vi "LDA_Align_PN_8 point.vi"(1 "Align Probe Using":enum16{"Green Beams", "Blue Beams"}(ring), 2 "Use Specification Beam Half-Angle":bool) -> (0 "Beam Data":T2={"Vg1 (Green 1 dir. vect.)"=[0.059117350659853476, -0.996541267827751, 0.05840068807144843], "Vg2  (Green 2 dir. vect.)"=[-0.05232536310393669, -0.9971561380468801, -0.054237373935992664], "Vb1 (Blue 1 dir. vect.)"=[-0.052923229613528855, -0.9969242065933935, 0.057803616456121795], "Vb2 (Blue 1 dir. vect.)"=[0.05971521716944564, -0.9967731992812374, -0.05364030232066602], "Porb (Orb XYZ posn. forced coplanar)"=[2201.0738225655555, -1199.3737231995547, 269.758310600838], "Porb (Orb XYZ posn. - allow skew)"=[2200.796256301178, -1199.3740953152687, 270.0329332816893], "Orb posn. uncertainty, +/- dx, dy, dz"=[0.13878313218879157, 0.00018605785703584843, 0.13731134042564008], "Vp (Actual Probe dir. vect)"=[0.003406702197773746, -0.9999920168246164, 0.0020882210543692924], "Yaw (deg)"=89.80480953887573, "Pitch (deg)"=0.11964634006213794, "In-Plane Roll (deg)"=45.305328966424156, "Beam Half Angle (deg)"=4.544091484248422, "B1 Close P11"=[0.0, 0.0, 0.0], "B1 Far P12"=[2158.01, -491.04, 229.28], "B2 Close P22"=[2158.01, -491.04, 229.28], "B2 Far P21"=[2158.01, -491.04, 229.28], "Projected Roll (deg)"=0.0, "Green Velocity Vector"=[0.0, 0.0, 0.0], "Blue Velocity Vector"=[0.0, 0.0, 0.0], "Probe is facing...."="-", "Calculation Method"=""} {"Vp (Actual Probe dir. vect)" format="%#_6f"; "Vg2  (Green 2 dir. vect.)" format="%#_6f"; "Vg1 (Green 1 dir. vect.)" format="%#_6f"})   [LabVIEW 2012]
uses:
  Controls/LDA_Beam_Cluster.ctl
  Gen Trav/Route mapping/Axis.ctl
  Controls/Tunnel_Coordinates.ctl
  Controls/Post_Process.ctl
  Controls/Setup.ctl
  Gen Trav/Trav_mode.ctl
  Controls/User_Specific_mode.ctl
  Globals/LDA_meas_global_1.vi
  Globals/Trav_pos_global.vi
panel:
  out "8 Peaked positions":dbl[][](array[numeric])
  out "Peakup up inputs":dbl[][](array[numeric])
  out "Fixed Axis":T1
  out "png folder":path
  out "Taught point names":string[](array[string])
  out "Taught Positions":dbl[][](array[numeric])
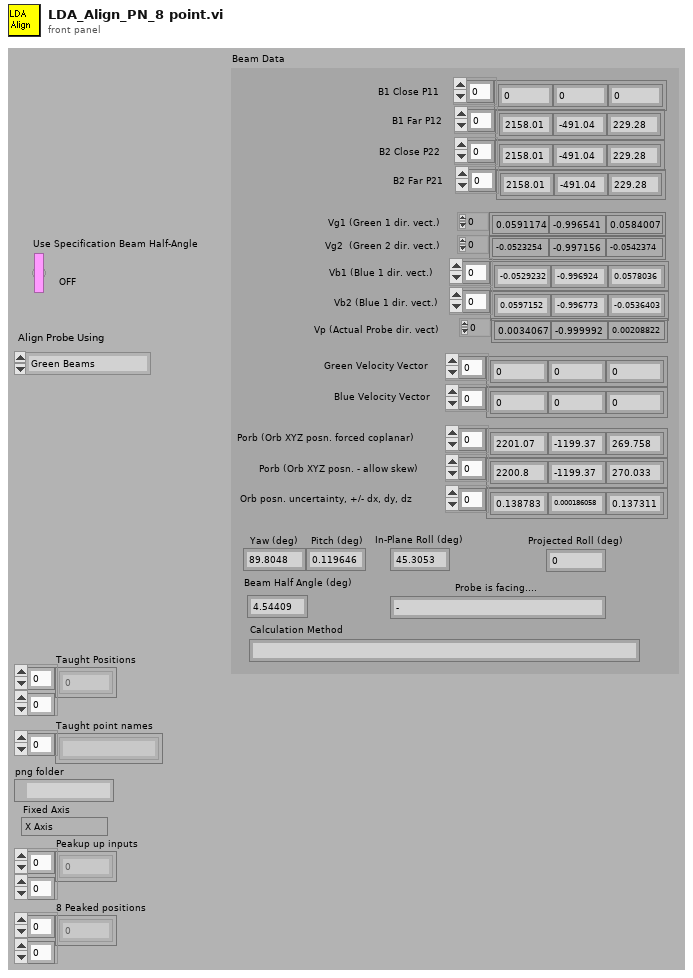
[diagram p1: front panel]
types:
  T1 = typedef "Axis.ctl" = enum16{"X Axis", "X Axis -ve", "Y Axis", "Y Axis -ve", "Z Axis", "Z Axis -ve"}
  T2 = typedef "LDA_Beam_Cluster.ctl" = cluster{"Vg1 (Green 1 dir. vect.)":dbl[], "Vg2  (Green 2 dir. vect.)":dbl[], "Vb1 (Blue 1 dir. vect.)":dbl[], "Vb2 (Blue 1 dir. vect.)":dbl[], "Porb (Orb XYZ posn. forced coplanar)":dbl[], "Porb (Orb XYZ posn. - allow skew)":dbl[], "Orb posn. uncertainty, +/- dx, dy, dz":dbl[], "Vp (Actual Probe dir. vect)":dbl[], "Yaw (deg)":dbl, "Pitch (deg)":dbl, "In-Plane Roll (deg)":dbl, "Beam Half Angle (deg)":dbl, "B1 Close P11":dbl[], "B1 Far P12":dbl[], "B2 Close P22":dbl[], "B2 Far P21":dbl[], "Projected Roll (deg)":dbl, "Green Velocity Vector":dbl[], "Blue Velocity Vector":dbl[], "Probe is facing....":string, "Calculation Method":string}
  T3 = typedef "Tunnel_Coordinates.ctl" = enum16{"Work in Tunnel Coordinates", "Work in Model Coordinates"}
  T4 = typedef "Setup.ctl" = enum16{"Run Program", "Show Setup", "Save Current Setup", "Setup Front Panel"}
  T5 = typedef "Post_Process.ctl" = enum16{"Take New Data", "Post Process Raw Data File"}
  T6 = typedef "User_Specific_mode.ctl" = enum16{"Check VI only", "Run VI"}
  T7 = typedef "Trav_mode.ctl" = enum16{"Move traverse", "Read traverse position", "Teach Position"}
  T8 = enum16{"Load setup from excel file", "Save setup to excel file"}
  T9 = cluster{"second":i32, "minute":i32, "hour":i32, "day of month":i32, "month":i32, "year":i32, "day of week":i32, "day of year":i32, "is DST":i32}
  T10 = typedef "Multi_Run_Status.ctl" = enum16{"Continue", "Jump to Next Point", "Jump to Next Row", "Jump To Fall Back", "Terminate Run"}
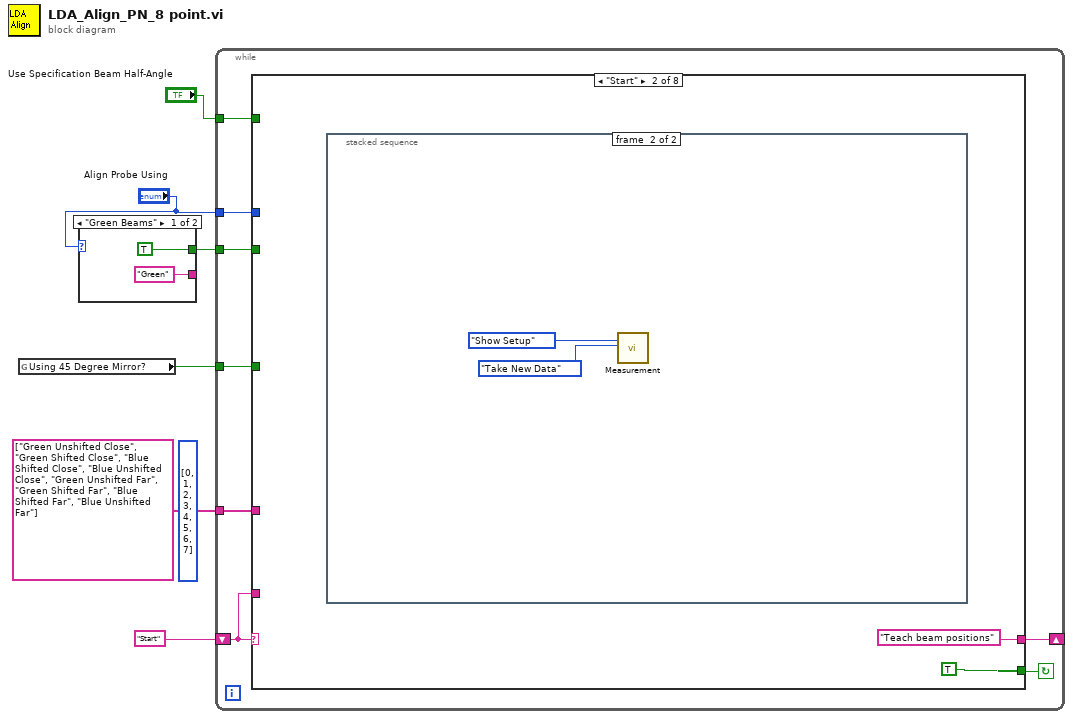
[diagram p0: block diagram]
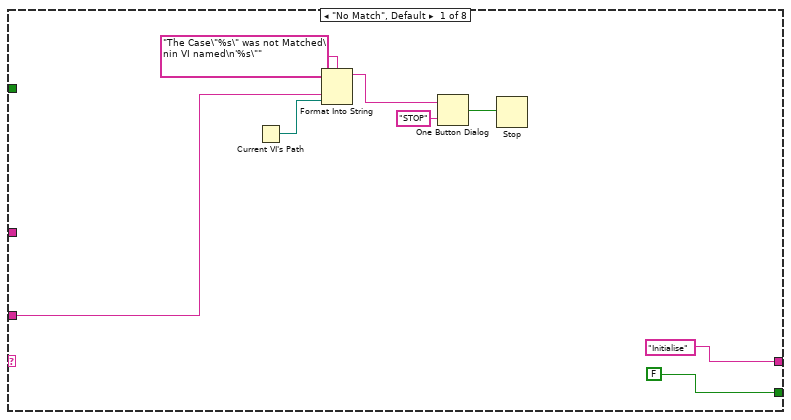
[diagram p2: hidden frame]
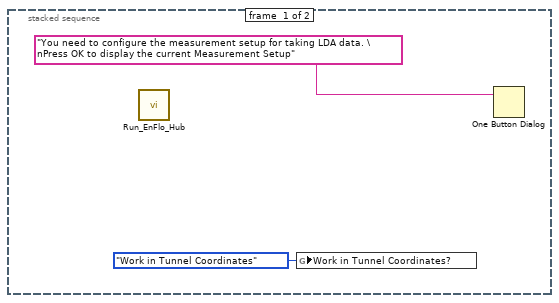
[diagram p3: hidden frame]
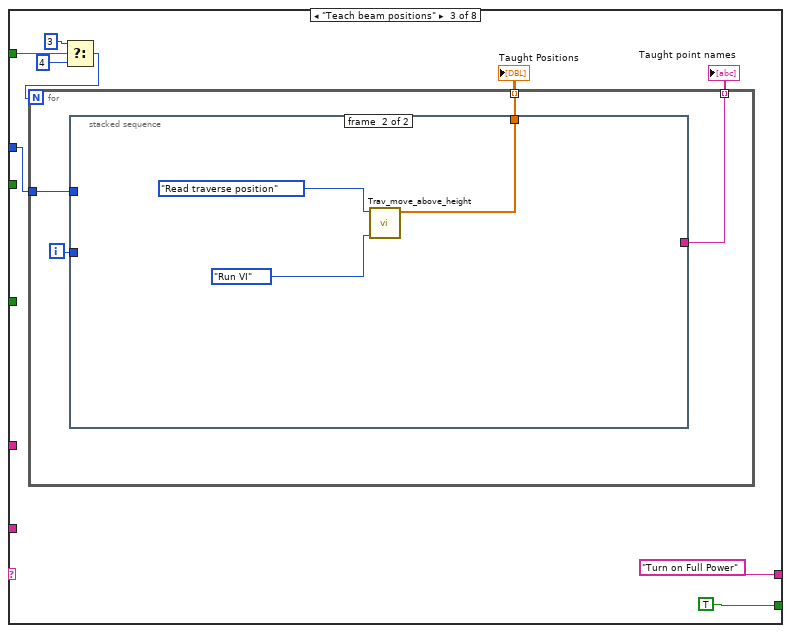
[diagram p4: hidden frame]
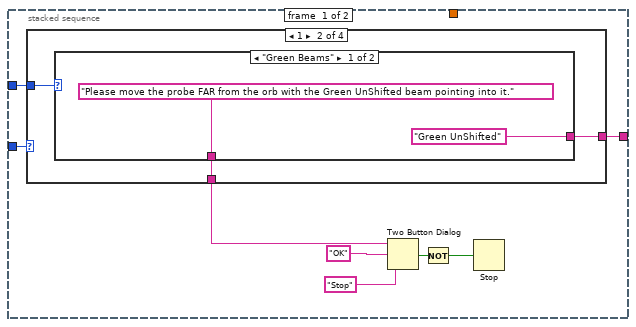
[diagram p5: hidden frame]
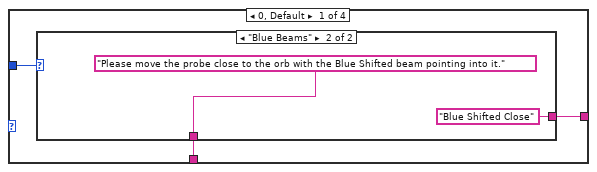
[diagram p6: hidden frame]
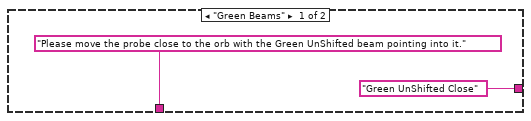
[diagram p7: hidden frame]
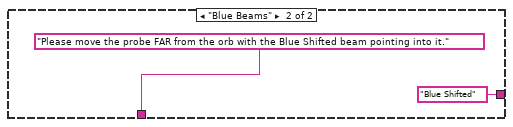
[diagram p8: hidden frame]
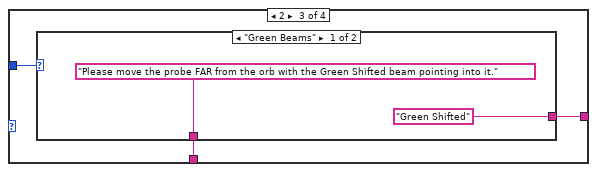
[diagram p9: hidden frame]
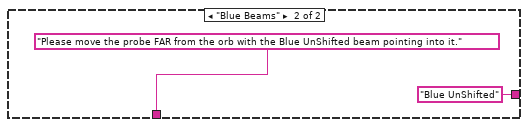
[diagram p10: hidden frame]
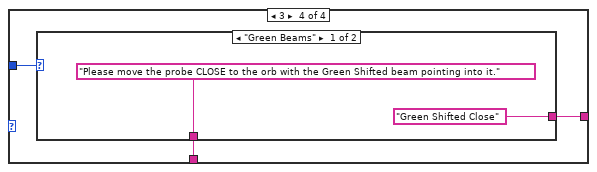
[diagram p11: hidden frame]
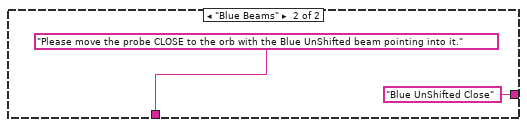
[diagram p12: hidden frame]
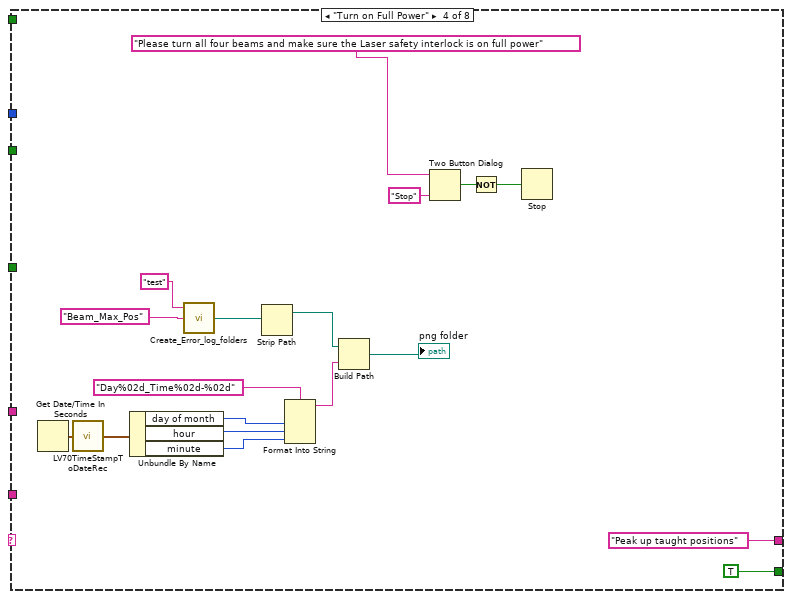
[diagram p13: hidden frame]
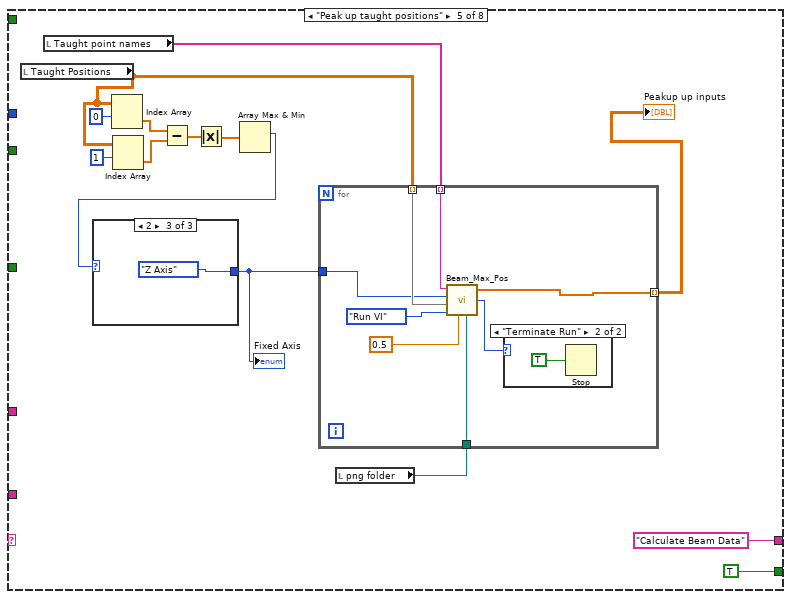
[diagram p14: hidden frame]
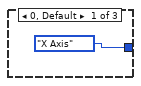
[diagram p15: hidden frame]
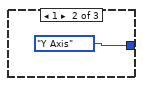
[diagram p16: hidden frame]
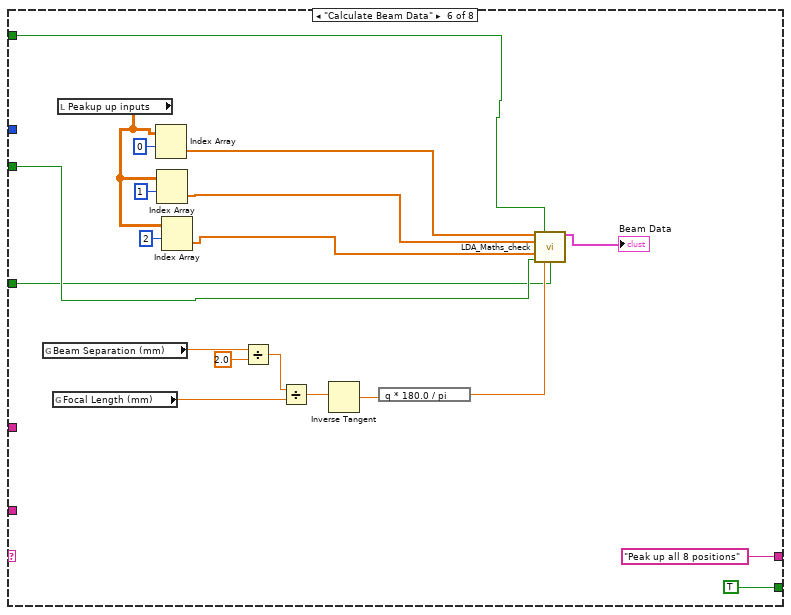
[diagram p18: hidden frame]
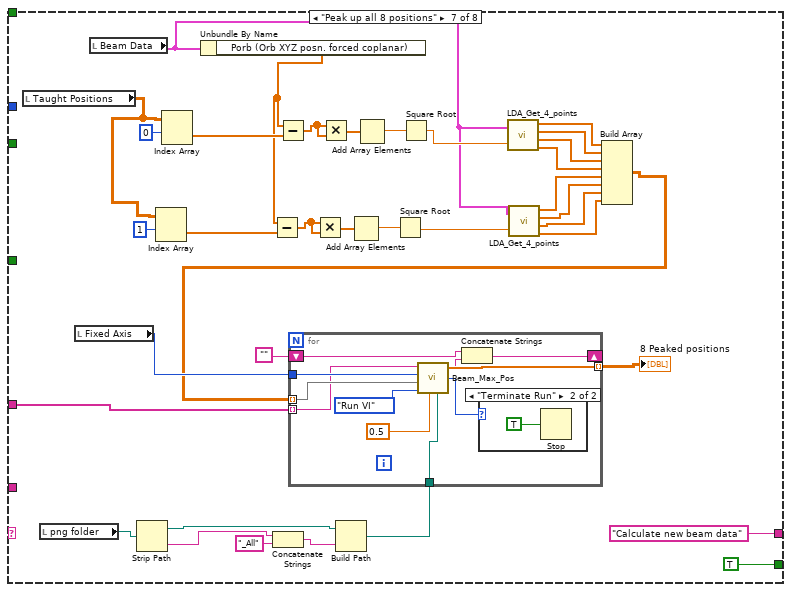
[diagram p19: hidden frame]
diagram:
  (unwired) i32[] [0, 1, 2, 3, 4, 5, 6, 7] ("appended array")
  n1 = global read "LDA_meas_global_1.vi" "Using 45 Degree Mirror?"() -> (w1:bool)
  n2 = case shown="\"Green Beams\"" "Align Probe Using" {
    tunnel: [TRUE FALSE] -> w3
    tunnel: ["Green" "Blue"] -> _
    frame "Green Beams" {
    }
    frame "Blue Beams" {
    }
  }
  n3 = while {
    shift-left: "Start" -> [w16]
    shift-right: [w17] -> _
    tunnel: "Align Probe Using" -> [w15]
    tunnel: "Use Specification Beam Half-Angle" -> [w14]
    tunnel: w3 -> [w13]
    tunnel: string[] ["Green Unshifted Close", "Green Shifted Close", "Blue Shifted Close", "Blue Unshifted Close", "Green Unshifted Far", "Green Shifted Far", "Blue Shifted Far", "Blue Unshifted Far"] ("appended array") -> [w12]
    tunnel: w1 -> [w11]
    stop <- w18 continue-if-true
    n4 = case shown="\"Start\"" w16 {
      tunnel: [FALSE TRUE TRUE TRUE TRUE TRUE TRUE FALSE] -> w18
      tunnel: ["Initialise" "Teach beam positions" "Turn on Full Power" "Peak up taught positions" "Calculate Beam Data" "Peak up all 8 positions" "Calculate new beam data" "Log Check Angles panel"] -> w17
      tunnel: w16 -> [w21 _ _ _ _ _ _ _]
      tunnel: w15 -> [_ _ w39 _ _ _ _ _]
      tunnel: w14 -> [_ _ w36 _ _ w146 _ _]
      tunnel: w13 -> [_ _ _ _ _ w145 _ _]
      tunnel: w12 -> [_ _ _ _ _ _ w151 _]
      tunnel: w11 -> [_ _ _ _ _ w129 _ w197]
      frame "No Match", Default {
        n5 = Current VI's Path() -> (path=w20:path)
        n6 = Format Into String(format string="The Case\"%s\" was not Matched\nin VI named\n'%s\"" ("Format String"), w21, w20) -> (resulting string=w24:string)  [unwired: 2 in, 1 out]
        n7 = One Button Dialog(message=w24, button name ("OK")="STOP") -> (true=w22:bool)
        n8 = Stop(stop? (T)=w22) -> ()
      }
      frame "Start" {
        n9 = stacked-sequence {
          frame #0 {
            n10 = call "Run_EnFlo_Hub.vi"() -> ()  [unwired: 8 out]
            n11 = global write "Trav_pos_global.vi" "Work in Tunnel Coordinates?"(Tunnel_Coordinates."Work in Tunnel Coordinates" ("Work in Tunnel Coordinates?")) -> ()
            n12 = One Button Dialog(message="You need to configure the measurement setup for taking LDA data. \nPress OK to display the current Measurement Setup") -> ()  [unwired: 1 in, 1 out]
          }
          frame #1 {
            n13 = call "Measurement.vi"("setup"=Setup."Show Setup", "Post Process"=Post_Process."Take New Data") -> ()  [unwired: 16 in, 2 out]
          }
        }
      }
      frame "Teach beam positions" {
        n14 = Select(t=3, s=w36, f=4) -> (s? t:f=w35:i32)
        n15 = for {
          N: w35 -> [_]
          tunnel: [w45] -> w34 mode=indexing
          tunnel: w39 -> [w44]
          tunnel: [w43] -> w33 mode=indexing
          i -> [w42]
          n16 = stacked-sequence {
            tunnel: [_ w82] -> w45
            tunnel: w44 -> [w52 _]
            tunnel: [w47 _] -> w43
            tunnel: w42 -> [w46 _]
            frame #0 {
              n17 = case shown="1" w46 {
                tunnel: [w56 w63 w70 w77] -> w53
                tunnel: w52 -> [w55 w62 w69 w76]
                tunnel: [w54 w61 w68 w75] -> w47
                frame 0, Default {
                  n18 = case shown="\"Blue Beams\"" w55 {
                    tunnel: ["Please move the probe close to the orb with the Green UnShifted beam pointing into it." ("message") "Please move the probe close to the orb with the Blue Shifted beam pointing into it." ("message")] -> w56
                    tunnel: ["Green UnShifted Close" "Blue Shifted Close"] -> w54
                    frame "Green Beams" {
                    }
                    frame "Blue Beams" {
                    }
                  }
                }
                frame 1 {
                  n19 = case shown="\"Green Beams\"" w62 {
                    tunnel: ["Please move the probe FAR from the orb with the Green UnShifted beam pointing into it." ("message") "Please move the probe FAR from the orb with the Blue Shifted beam pointing into it." ("message")] -> w63
                    tunnel: ["Green UnShifted" "Blue Shifted"] -> w61
                    frame "Green Beams" {
                    }
                    frame "Blue Beams" {
                    }
                  }
                }
                frame 2 {
                  n20 = case shown="\"Green Beams\"" w69 {
                    tunnel: ["Please move the probe FAR from the orb with the Green Shifted beam pointing into it." ("message") "Please move the probe FAR from the orb with the Blue UnShifted beam pointing into it." ("message")] -> w70
                    tunnel: ["Green Shifted" "Blue UnShifted"] -> w68
                    frame "Green Beams" {
                    }
                    frame "Blue Beams" {
                    }
                  }
                }
                frame 3 {
                  n21 = case shown="\"Green Beams\"" w76 {
                    tunnel: ["Please move the probe CLOSE to the orb with the Green Shifted beam pointing into it." ("message") "Please move the probe CLOSE to the orb with the Blue UnShifted beam pointing into it." ("message")] -> w77
                    tunnel: ["Green Shifted Close" "Blue UnShifted Close"] -> w75
                    frame "Green Beams" {
                    }
                    frame "Blue Beams" {
                    }
                  }
                }
              }
              n22 = Two Button Dialog(message=w53, 1:"Stop" ("F button name (\"Cancel\")"), 2:"OK" ("T button name (\"OK\")")) -> (T button?=w49:bool)
              n23 = Not(x=w49) -> (.not. x?=w48:bool)
              n24 = Stop(stop? (T)=w48) -> ()
            }
            frame #1 {
              n25 = call "Trav_move_above_height.vi"("Simulate/Run"=User_Specific_mode."Run VI", "Mode"=Trav_mode."Read traverse position") -> ("Trav Position achieved"=w82:dbl[])  [unwired: 5 in, 4 out]
            }
          }
        }
        "Taught Positions" <- w34
        "Taught point names" <- w33
      }
      frame "Turn on Full Power" {
        n26 = Get Date/Time In Seconds() -> (seconds since 1Jan1904=w85:timestamp)
        n27 = call <vilib>:"LV70TimeStampToDateRec.vi"("time stamp"=w85) -> ("date time rec"=w94:T9)
        n28 = Unbundle By Name(w94) -> ("day of month"=w91:i32, "hour"=w92:i32, "minute"=w93:i32)
        n29 = call "Create_Error_log_folders.vi"("Log Folder"="Beam_Max_Pos" ("name or relative path"), "Log Filename"="test") -> ("Server copy Location"=w86:path)  [unwired: 1 in, 2 out]
        n30 = Strip Path(path=w86) -> (stripped path=w95:path)  [unwired: 1 out]
        n31 = Format Into String(format string="Day%02d_Time%02d-%02d", w91, w92, w93) -> (resulting string=w96:string)  [unwired: 2 in, 1 out]
        n32 = Build Path(base path=w95, name or relative path=w96) -> (appended path=→"png folder":path)
        n33 = Two Button Dialog(message="Please turn all four beams and make sure the Laser safety interlock is on full power", 1:"Stop" ("F button name (\"Cancel\")")) -> (T button?=w100:bool)  [unwired: 1 out]
        n34 = Not(x=w100) -> (.not. x?=w101:bool)
        n35 = Stop(stop? (T)=w101) -> ()
      }
      frame "Peak up taught positions" {
        n36 = local read "Taught Positions"() -> (w107:dbl[][])
        n37 = local read "Taught point names"() -> (w106:string[])
        n38 = Index Array(array=w107, index (row)=0) -> (element=w110:dbl[])  [unwired: 1 in]
        n39 = Index Array(array=w107, index (row)=1) -> (element=w111:dbl[])  [unwired: 1 in]
        n40 = Subtract(x=w110, y=w111) -> (x-y=w112:dbl[])
        n41 = Absolute Value(x=w112) -> (abs(x)=w113:dbl[])
        n42 = Array Max & Min(array=w113) -> (max index (indices)=w114:i32)  [unwired: 3 out]
        n43 = case shown="2" w114 {
          tunnel: [Axis."X Axis" ("Fixed Axis") Axis."Y Axis" ("Fixed Axis") Axis."Z Axis" ("Fixed Axis")] -> w105
          frame 0, Default {
          }
          frame 1 {
          }
          frame 2 {
          }
        }
        "Fixed Axis" <- w105
        n44 = local read "png folder"() -> (w104:path)
        n45 = for {
          tunnel: w106 -> [w127] mode=indexing
          tunnel: w107 -> [w126] mode=indexing
          tunnel: w105 -> [w124]
          tunnel: w104 -> [w123]
          tunnel: [w122] -> w103 mode=indexing
          n46 = call "Beam_Max_Pos.vi"("Picture Log"=w123, "Search Step (mm)"=0.5, "Mode"=User_Specific_mode."Run VI", "Starting Position"=w126, "Fixed Axis"=w124, "Beam Name"=w127) -> ("Status"=w120:T10, "Beam maxima"=w122:dbl[])  [unwired: 1 in, 2 out]
          n47 = case shown="\"Terminate Run\"" w120 {
            frame "Continue", Default {
            }
            frame "Terminate Run" {
              n48 = Stop(stop? (T)=TRUE) -> ()
            }
          }
        }
        "Peakup up inputs" <- w103
      }
      frame "Calculate Beam Data" {
        n49 = global read "LDA_meas_global_1.vi" "Beam Separation (mm)"() -> (w132:dbl)
        n50 = global read "LDA_meas_global_1.vi" "Focal Length (mm)"() -> (w135:dbl)
        n51 = local read "Peakup up inputs"() -> (w138:dbl[][])
        n52 = Index Array(array=w138, index (row)=0) -> (element=w142:dbl[])  [unwired: 1 in]
        n53 = Index Array(array=w138, index (row)=1) -> (element=w143:dbl[])  [unwired: 1 in]
        n54 = Index Array(array=w138, index (row)=2) -> (element=w144:dbl[])  [unwired: 1 in]
        n55 = Divide(x=w132, y=2.0) -> (x/y=w134:dbl)
        n56 = Divide(x=w134, y=w135) -> (x/y=w137:dbl)
        n57 = Inverse Tangent(1:w137) -> (0:w136:dbl)
        n58 = expression code="q * 180.0 / pi"(w136) -> (w131:dbl)
        n59 = call "LDA_Maths_check.vi"("B1 Close P11"=w142, "Use Specification Beam Half-Angle"=w146, "B1 Far P12"=w143, "B2 Far P21"=w144, "Use Green Beams (True) or Blue Beams (False)"=w145, "Beam Half-Angle (deg)"=w131, "Using 45 Degree Mirror?"=w129) -> ("Beam Data"=→"Beam Data":T2)  [unwired: 8 out]
      }
      frame "Peak up all 8 positions" {
        n60 = local read "Taught Positions"() -> (w172:dbl[][])
        n61 = local read "png folder"() -> (w163:path)
        n62 = local read "Fixed Axis"() -> (w164:T1)
        n63 = local read "Beam Data"() -> (w170:T2)
        n64 = Strip Path(path=w163) -> (stripped path=w159:path, name=w162:string)
        n65 = Index Array(array=w172, index (row)=1) -> (element=w173:dbl[])  [unwired: 1 in]
        n66 = Index Array(array=w172, index (row)=0) -> (element=w182:dbl[])  [unwired: 1 in]
        n67 = Unbundle By Name(w170) -> ("Porb (Orb XYZ posn. forced coplanar)"=w150:dbl[])
        n68 = Subtract(x=w150, y=w173) -> (x-y=w177:dbl[])
        n69 = Concatenate Strings(w162, "_All" ("string")) -> (w160:string)
        n70 = Subtract(x=w150, y=w182) -> (x-y=w178:dbl[])
        n71 = Multiply(x=w177, y=w177) -> (x*y=w176:dbl[])
        n72 = Multiply(x=w178, y=w178) -> (x*y=w179:dbl[])
        n73 = Build Path(base path=w159, name or relative path=w160) -> (appended path=w149:path)
        n74 = Add Array Elements(numeric array=w176) -> (sum=w175:dbl)
        n75 = Add Array Elements(numeric array=w179) -> (sum=w180:dbl)
        n76 = Square Root(x=w175) -> (sqrt(x)=w169:dbl)
        n77 = Square Root(x=w180) -> (sqrt(x)=w171:dbl)
        n78 = call "LDA_Get_4_points.vi"("Beam Data"=w170, "L, Probe-Normal Distance"=w171) -> ("Pg1"=w168:dbl[], "Pg2"=w167:dbl[], "Pb1"=w166:dbl[], "Pb2"=w165:dbl[])
        n79 = call "LDA_Get_4_points.vi"("Beam Data"=w170, "L, Probe-Normal Distance"=w169) -> ("Pg1"=w156:dbl[], "Pg2"=w155:dbl[], "Pb1"=w157:dbl[], "Pb2"=w158:dbl[])
        n80 = Build Array(w168, w167, w166, w165, w156, w155, w157, w158) -> (w154:dbl[][])
        n81 = for {
          tunnel: w149 -> [w194]
          tunnel: [w193] -> w152 mode=indexing
          shift-right: [w190] -> _
          shift-left: "" -> [w192]
          tunnel: w154 -> [w187] mode=indexing
          tunnel: w164 -> [w186]
          tunnel: w151 -> [w185] mode=indexing
          n82 = call "Beam_Max_Pos.vi"("Picture Log"=w194, "Search Step (mm)"=0.5, "Mode"=User_Specific_mode."Run VI", "Starting Position"=w187, "Fixed Axis"=w186, "Beam Name"=w185) -> ("Status"=w188:T10, "Beam maxima"=w193:dbl[], "Message"=w191:string)  [unwired: 1 in, 1 out]
          n83 = Concatenate Strings(w192, w191) -> (w190:string)
          n84 = case shown="\"Terminate Run\"" w188 {
            frame "Continue", Default {
            }
            frame "Terminate Run" {
              n85 = Stop(stop? (T)=TRUE) -> ()
            }
          }
        }
        "8 Peaked positions" <- w152
      }
      frame "Calculate new beam data" {
        w210 = FALSE  # Use Green Beams (True) or Blue Beams (False)
        w227 = TRUE  # Use Green Beams (True) or Blue Beams (False)
        n86 = local read "8 Peaked positions"() -> (w208:dbl[][])
        n87 = Index Array(array=w208, index (row)=7) -> (element=w218:dbl[])  [unwired: 1 in]
        n88 = Index Array(array=w208, index (row)=3) -> (element=w217:dbl[])  [unwired: 1 in]
        n89 = Index Array(array=w208, index (row)=5) -> (element=w219:dbl[])  [unwired: 1 in]
        n90 = Index Array(array=w208, index (row)=6) -> (element=w216:dbl[])  [unwired: 1 in]
        n91 = Index Array(array=w208, index (row)=1) -> (element=w220:dbl[])  [unwired: 1 in]
        n92 = Index Array(array=w208, index (row)=4) -> (element=w221:dbl[])  [unwired: 1 in]
        n93 = Index Array(array=w208, index (row)=2) -> (element=w212:dbl[])  [unwired: 1 in]
        n94 = Index Array(array=w208, index (row)=0) -> (element=w225:dbl[])  [unwired: 1 in]
        n95 = call "LDA_Maths_check.vi"("B1 Close P11"=w212, "Use Specification Beam Half-Angle"=FALSE, "B1 Far P12"=w216, "B2 Close P22"=w217, "B2 Far P21"=w218, "Use Green Beams (True) or Blue Beams (False)"=w210, "Using 45 Degree Mirror?"=w197) -> ("Beam Data"=w198:T2)  [unwired: 1 in, 7 out]
        n96 = call "LDA_Maths_check.vi"("B1 Close P11"=w225, "Use Specification Beam Half-Angle"=FALSE, "B1 Far P12"=w221, "B2 Close P22"=w220, "B2 Far P21"=w219, "Use Green Beams (True) or Blue Beams (False)"=w227, "Using 45 Degree Mirror?"=w197) -> ("Beam Data"=w201:T2)  [unwired: 1 in, 7 out]
        n97 = Unbundle By Name(w201) -> ("Vg1 (Green 1 dir. vect.)"=w207:dbl[], "Vg2  (Green 2 dir. vect.)"=w206:dbl[])
        n98 = Unbundle By Name(w198) -> ("Vb1 (Blue 1 dir. vect.)"=w205:dbl[], "Vb2 (Blue 1 dir. vect.)"=w204:dbl[])
        n99 = call "Read_Write_Beam_Data.vi"("Beam Data In"=w198, "Mode"=T8."Save setup to excel file") -> ()  [unwired: 1 out]
        n100 = call "Read_Write_Beam_Data.vi"("Beam Data In"=w201, "Mode"=T8."Save setup to excel file") -> ()  [unwired: 1 out]
        n101 = call "LDA_Angle_Checks.vi"("Vg1"=w207, "Vg2"=w206, "Vb1"=w205, "Vb2"=w204) -> ()  [unwired: 16 out]
      }
    }
  }
